vi "getState.vi"(8 "error in (no error)":errorcluster, 11 "Memento in":refnum<class "Memento.lvclass">) -> (0 "error out":errorcluster, 2 "State":string, 3 "Memento out":refnum<class "Memento.lvclass">)   [LabVIEW 2016, in "Memento.lvclass"]
uses:
  Memento.lvclass
  Memento.lvclass/Memento.ctl
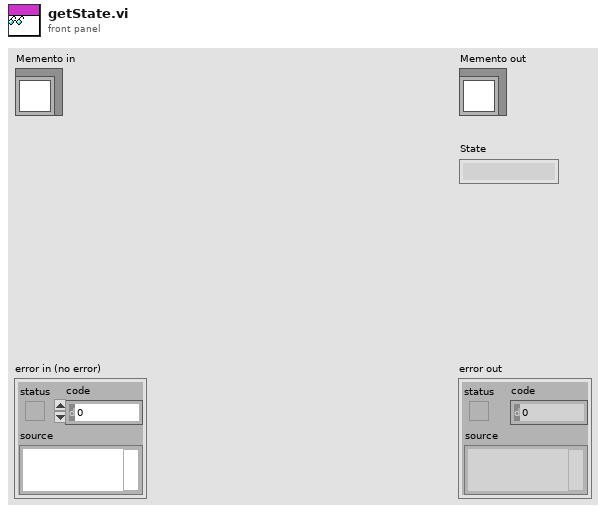
[diagram p1: front panel]
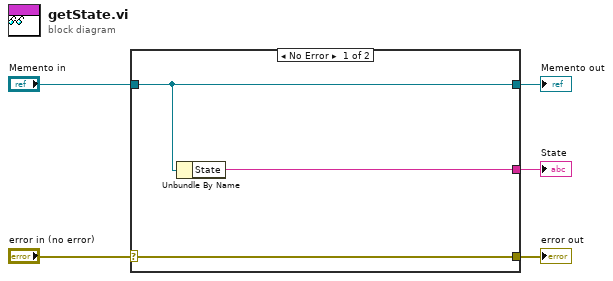
[diagram p0: block diagram]
diagram:
  n1 = case shown="No Error" "error in (no error)" {
    selector: "error in (no error)" -> [w8 w9]
    tunnel: [w8 w9] -> w4
    tunnel: [w7 w10] -> w2
    tunnel: "Memento in" -> [w7 w10]
    tunnel: [w6 _] -> w1
    frame No Error {
      n2 = Unbundle By Name(w7) -> ("State"=w6:string)
    }
    frame Error {
    }
  }
  "error out" <- w4
  "Memento out" <- w2
  "State" <- w1
